vi "support.read_and_free_array_multiline_string_at_address.vi"(6 "string length":u64, 8 "error in (no error)":errorcluster, 11 "table_names_ptr":u64) -> (0 "error out":errorcluster, 3 "lines":string[](array[string]))   [LabVIEW 2020, in "reqwest.lvlib"]
uses:
  reqwest.lvlib
  <userlib>/_OpenG.lib/string/string.llb/openg_string.lvlib
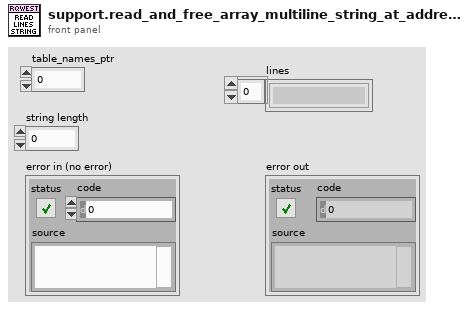
[diagram p1: front panel]
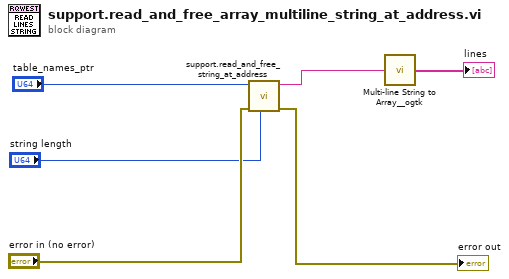
[diagram p0: block diagram]
diagram:
  n1 = call "support.read_and_free_string_at_address.vi"("string_length"="string length", "error in (no error)"="error in (no error)", "string_ptr"="table_names_ptr") -> ("error out"=→"error out":errorcluster, "string"=w2:string)  [unwired: 7 in]
  n2 = call <userlib>:"Multi-line String to Array__ogtk.vi"("string"=w2) -> ("lines"=→"lines":string[])
